vi "SQLite Get Fields Info v2.vi"(8 "error in":errorcluster, 10 "Table Name":string="test", 11 "SQLite Connection":refnum<class "Connection.lvclass">) -> (0 "error out":errorcluster, 2 "Fields Info":T1[](array[typedef]), 3 "Dup SQLite Connection":refnum<class "Connection.lvclass">)   [LabVIEW 2021, in "EDT SQLite+.lvlib"]
uses:
  EDT SQLite+.lvlib
  SQLite Field Info.ctl
  SQLite Data Type.ctl
  <vilib>/drjdpowell/SQLite Library/SQL Connection/Connection.lvclass
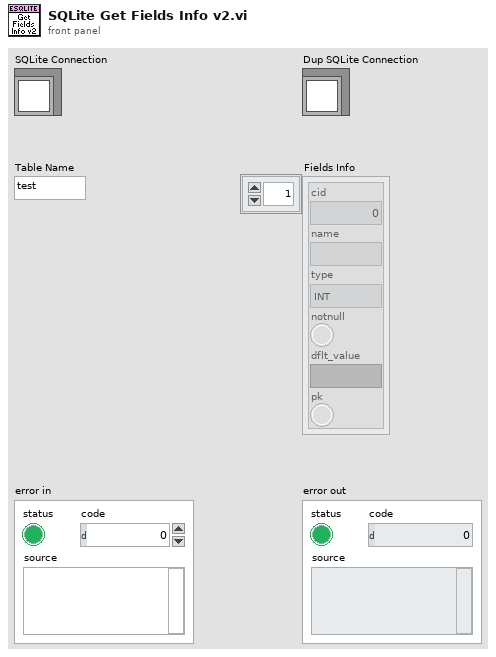
[diagram p1: front panel]
types:
  T1 = typedef "EDT SQLite+.lvlib/SQLite Field Info.ctl" = cluster{"cid":i32, "name":string, "type":T2, "notnull":bool, "dflt_value":variant, "pk":bool}
  T2 = typedef "EDT SQLite+.lvlib/SQLite Data Type.ctl" = enum16{"INT", "INTEGER", "TINYINT", "SMALLINT", "MEDIUMINT", "BIGINT", "UNSIGNED BIG INT", "INT2", "INT8", "CHARACTER", "VARCHAR", "VARYING CHARACTER", "NCHAR", "NATIVE CHARACTER", "NVARCHAR", "TEXT", "CLOB", "BLOB", "no datatype specified", "REAL", "DOUBLE", "DOUBLE PRECISION", "FLOAT", "NUMERIC", "DECIMAL", "BOOLEAN", "DATE", "DATETIME"}
  T3 = typedef "EDT SQLite+.lvlib/SQLite Foreign Key.ctl" = cluster{"id":i64, "seq":i64, "table":string, "from":string, "to":string, "on_update":T4, "on_delete":T4, "match":T4}
  T4 = typedef "EDT SQLite+.lvlib/SQLite Reaction Type.ctl" = enum16{"NO ACTION", "SET NULL", "SET DEFAULT", "CASCADE", "RESTRICT", "NONE"}
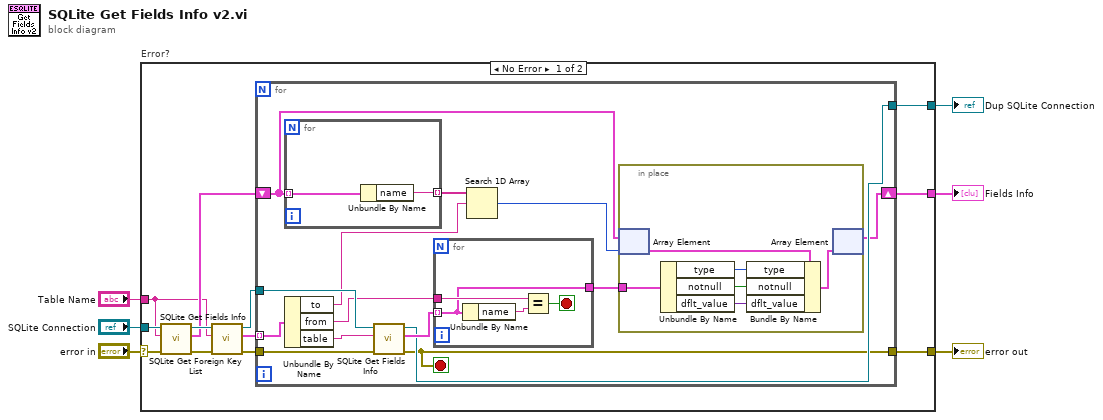
[diagram p0: block diagram]
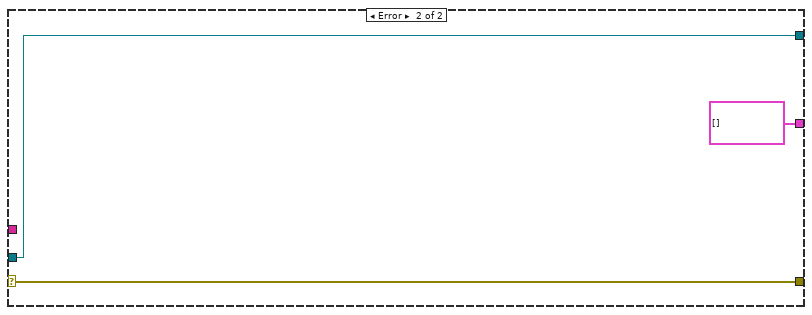
[diagram p2: hidden frame]
diagram:
  n1 = case "Error?" shown="No Error" "error in" {
    selector: "error in" -> [w17 w47]
    tunnel: "Table Name" -> [w7 _]
    tunnel: [w10 T1[] []] -> w3
    tunnel: [w8 w47] -> w4
    tunnel: "SQLite Connection" -> [w18 w45]
    tunnel: [w9 w45] -> w1
    frame No Error {
      n2 = call "SQLite Get Fields Info.vi"("error in"=w17, "Table Name"=w7, "SQLite Connection"=w18) -> ("error out"=w15:errorcluster, "Fields Info"=w11:T1[], "Dup SQLite Connection"=w16:refnum<class "Connection.lvclass">)  [unwired: 6 in]
      n3 = call "SQLite Get Foreign Key List.vi"("error in"=w15, "Table Name"=w7, "SQLite Connection"=w16) -> ("error out"=w12:errorcluster, "Foreign Key List"=w14:T3[], "Dup SQLite Connection"=w13:refnum<class "Connection.lvclass">)  [unwired: 6 in]
      n4 = for {
        tunnel: w14 -> [w32] mode=indexing
        tunnel: w13 -> [w31]
        tunnel: w12 -> [w30]
        shift-right: [w22] -> w10
        shift-left: w11 -> [w21]
        tunnel: [w26] -> w9
        tunnel: [w25] -> w8
        stop <- w25 stop-if-true
        n5 = for {
          tunnel: w21 -> [w40] mode=indexing
          tunnel: [w39] -> w27 mode=indexing
          n6 = Unbundle By Name(w40) -> ("name"=w39:string)
        }
        n7 = Unbundle By Name(w32) -> ("to"=w23:string, "from"=w28:string, "table"=w24:string)
        n8 = call "SQLite Get Fields Info.vi"("error in"=w30, "Table Name"=w24, "SQLite Connection"=w31) -> ("error out"=w25:errorcluster, "Fields Info"=w29:T1[], "Dup SQLite Connection"=w26:refnum<class "Connection.lvclass">)  [unwired: 6 in]
        n9 = for {
          tunnel: w29 -> [w41] mode=indexing
          tunnel: w28 -> [w43]
          tunnel: [w41] -> w19
          stop <- w42 stop-if-true
          n10 = Unbundle By Name(w41) -> ("name"=w44:string)
          n11 = Equal?(x=w43, y=w44) -> (x = y?=w42:bool)
        }
        n12 = Search 1D Array(1D array=w27, element=w23) -> (index of element=w20:i32)  [unwired: 1 in]
        n13 = in-place {
          in-place-border: w19 -> [w36]
          n14 = in-place-array #1(w21, w20) -> (w38:T1)
          n15 = Unbundle By Name(w36) -> ("type"=w35:T2, "notnull"=w34:bool, "dflt_value"=w33:variant)
          n16 = Bundle By Name(cluster=w38, "type"=w35, "notnull"=w34, "dflt_value"=w33) -> (w37:T1)
          n17 = in-place-array #1(w37) -> (w22:T1[])  [unwired: 1 out]
        }
      }
    }
    frame Error {
    }
  }
  "error out" <- w4
  "Fields Info" <- w3
  "Dup SQLite Connection" <- w1
